vi "Convert_Version_Info.vi"(8 "error in (no error)":errorcluster, 11 "AB_Targetfile in":refnum<class "AB_Targetfile.lvclass">) -> (0 "error out":errorcluster, 2 "input version info":T1={"PrivateBuild"="", "SpecialBuild"="", "LegalCopyright"="", "LegalTrademarks"="", "Comments"="", "FileDescription"="", "InternalName"="", "file version"={"major"=1, "minor"=0, "patch"=0, "build"=0}, "ProductName"="", "FileType"=0, "CompanyName"="", "OriginalFilename"=""} {"FileType" items=["VFT_UNKNOWN", "VFT_APP", "VFT_DLL", "VFT_DRV", "VFT_FONT", "VFT_VXD", "-", "VFT_STATIC_LIB"]}, 3 "AB_Targetfile out":refnum<class "AB_Targetfile.lvclass">)   [LabVIEW 2020, in "AB_Targetfile.lvclass"]
uses:
  <vilib>/AppBuilder/AB_Classes/TargetFile/AB_Targetfile.lvclass
  <vilib>/AppBuilder/AB_Version_Info.ctl
  <vilib>/AppBuilder/AB_Classes/TargetFile/AB_Targetfile.lvclass/AB_Targetfile.ctl
  <vilib>/AppBuilder/AB_Classes/Build/AB_Build.lvclass
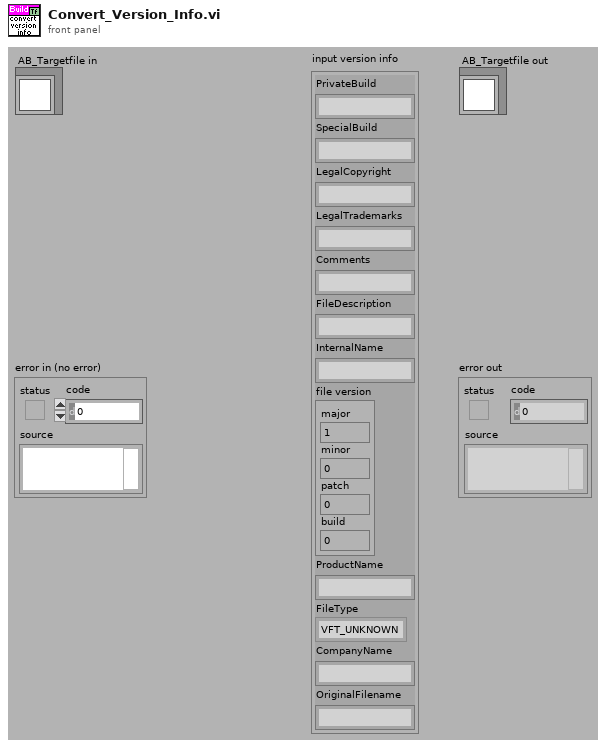
[diagram p1: front panel]
types:
  T1 = typedef "AB_Version_Info.ctl" = cluster{"PrivateBuild":string, "SpecialBuild":string, "LegalCopyright":string, "LegalTrademarks":string, "Comments":string, "FileDescription":string, "InternalName":string, "file version":cluster{"major":u16, "minor":u16, "patch":u16, "build":u16}, "ProductName":string, "FileType":u16, "CompanyName":string, "OriginalFilename":string}
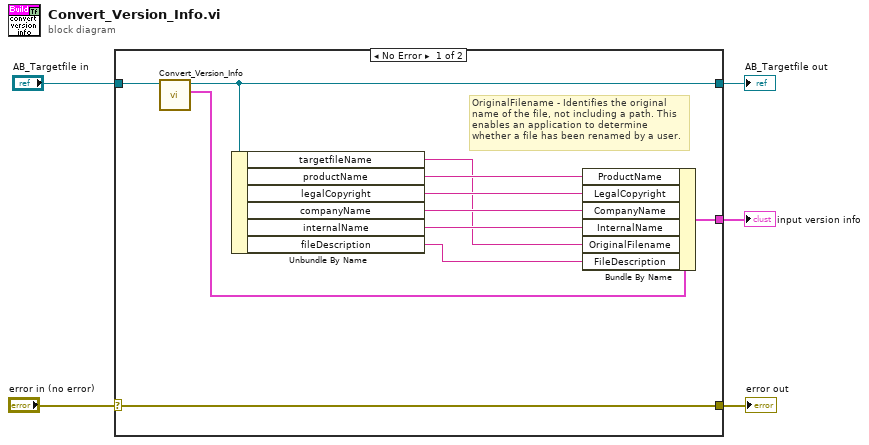
[diagram p0: block diagram]
diagram:
  n1 = case shown="No Error" "error in (no error)" {
    selector: "error in (no error)" -> [w16 w18]
    tunnel: [w16 w18] -> w4
    tunnel: [w7 w17] -> w2
    tunnel: "AB_Targetfile in" -> [w8 w17]
    tunnel: [w10 _] -> w1
    frame No Error {
      # "OriginalFilename - Identifies the original name of the file, not including a path. This enables an application to determine whether a file has been renamed by a user."
      n2 = call-parent "Convert_Version_Info.vi"("AB_Build in"=w8) -> ("input version info"=w6:T1, "AB_Build out"=w7:refnum<class "AB_Targetfile.lvclass">)  [unwired: 8 in, 1 out]
      n3 = Unbundle By Name(w7) -> ("targetfileName"=w9:string, "productName"=w15:string, "legalCopyright"=w14:string, "companyName"=w13:string, "internalName"=w12:string, "fileDescription"=w11:string)
      n4 = Bundle By Name(cluster=w6, "ProductName"=w15, "LegalCopyright"=w14, "CompanyName"=w13, "InternalName"=w12, "OriginalFilename"=w9, "FileDescription"=w11) -> (w10:T1)
    }
    frame Error {
    }
  }
  "error out" <- w4
  "AB_Targetfile out" <- w2
  "input version info" <- w1
